vi "Timer data class VI - timer interface.vi"(8 "error in (no error)":errorcluster, 11 "Timer in":refnum<class "Timer.lvclass">) -> (0 "error out":errorcluster, 1 "counter":i8, 2 "time":string, 3 "Timer out":refnum<class "Timer.lvclass">, 5 "Milliseconds":u32)   [LabVIEW 2010, in "Timer.lvclass"]
uses:
  Timer.lvclass
  Controls/Timing Control.ctl
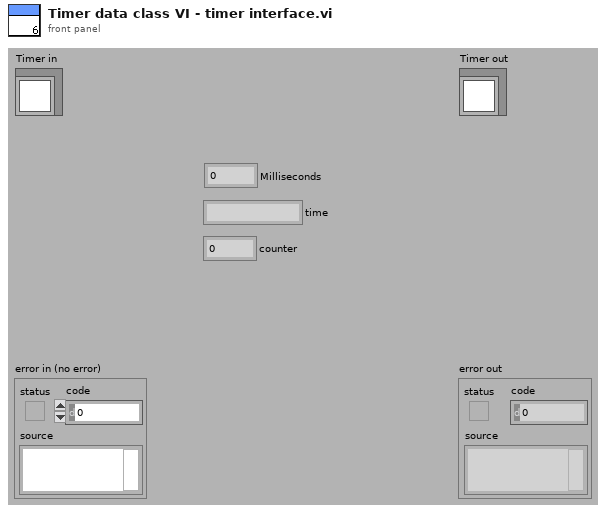
[diagram p1: front panel]
types:
  T1 = typedef "Timing Control.ctl" = enum16{"Idle", "Start", "Continue", "Reset"}
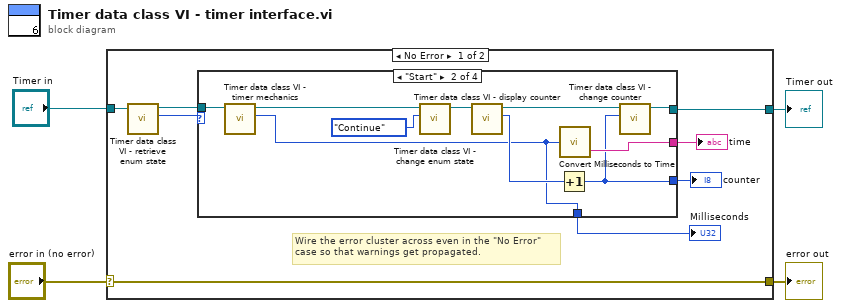
[diagram p0: block diagram]
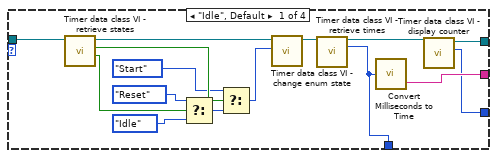
[diagram p2: hidden frame]
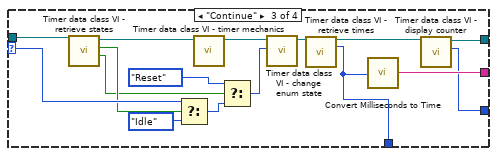
[diagram p3: hidden frame]
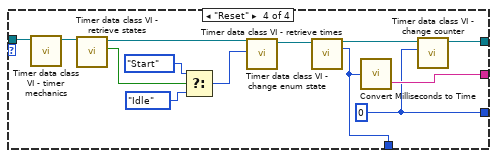
[diagram p4: hidden frame]
diagram:
  n1 = case shown="No Error" "error in (no error)" {
    selector: "error in (no error)" -> [w12 w68]
    tunnel: [w12 w68] -> w3
    tunnel: [w7 w67] -> w1
    tunnel: "Timer in" -> [w11 w67]
    frame No Error {
      # "Wire the error cluster across even in the \"No Error\"\ncase so that warnings get propagated."
      n2 = call-dynamic "Timer data class VI - retrieve enum state.vi"("Timer in"=w11) -> ("State"=w10:T1, "Timer out"=w9:refnum<class "Timer.lvclass">)  [unwired: 8 in, 1 out]
      n3 = case shown="\"Start\"" w10 {
        selector: w10 -> [_ _ w45 _]
        tunnel: w9 -> [w26 w36 w53 w66]
        tunnel: [w27 w37 w42 w60] -> w8
        tunnel: [w15 w31 w40 w56] -> w7
        tunnel: [w14 w29 w39 w55] -> w6
        tunnel: [w13 w28 w38 w54] -> w5
        frame "Idle", Default {
          n4 = call-dynamic "Timer data class VI - retrieve states.vi"("Timer in"=w26) -> ("Reset"=w21:bool, "Start/Stop"=w20:bool, "Timer out"=w25:refnum<class "Timer.lvclass">)  [unwired: 7 in, 1 out]
          n5 = Select(t=Timing_Control."Reset" ("Enum"), s=w21, f=Timing_Control."Idle" ("Enum")) -> (s? t:f=w23:T1)
          n6 = Select(t=Timing_Control."Start" ("Enum"), s=w20, f=w23) -> (s? t:f=w22:T1)
          n7 = call-dynamic "Timer data class VI - change enum state.vi"("State"=w22, "Timer in"=w25) -> ("Timer out"=w24:refnum<class "Timer.lvclass">)  [unwired: 8 in, 1 out]
          n8 = call-dynamic "Timer data class VI - retrieve times.vi"("Timer in"=w24) -> ("Timer out"=w16:refnum<class "Timer.lvclass">, "Milliseconds"=w13:u32)  [unwired: 10 in, 3 out]
          n9 = call "Convert Milliseconds to Time.vi"("milliseconds"=w13) -> ("elapsed time"=w27:string)  [unwired: 1 in]
          n10 = call "Timer data class VI - display counter.vi"("Timer in"=w16) -> ("Counter"=w14:i8, "Timer out"=w15:refnum<class "Timer.lvclass">)  [unwired: 8 in, 1 out]
        }
        frame "Start" {
          n11 = call-dynamic "Timer data class VI - timer mechanics.vi"("Timer in"=w36) -> ("elapsed time (milliseconds)"=w28:u32, "Timer out"=w35:refnum<class "Timer.lvclass">)  [unwired: 8 in, 1 out]
          n12 = call-dynamic "Timer data class VI - change enum state.vi"("State"=Timing_Control."Continue" ("Enum"), "Timer in"=w35) -> ("Timer out"=w33:refnum<class "Timer.lvclass">)  [unwired: 8 in, 1 out]
          n13 = call "Timer data class VI - display counter.vi"("Timer in"=w33) -> ("Counter"=w30:i8, "Timer out"=w32:refnum<class "Timer.lvclass">)  [unwired: 8 in, 1 out]
          n14 = Increment(x=w30) -> (x+1=w29:i8)
          n15 = call "Convert Milliseconds to Time.vi"("milliseconds"=w28) -> ("elapsed time"=w37:string)  [unwired: 1 in]
          n16 = call "Timer data class VI - change counter.vi"("Counter"=w29, "Timer in"=w32) -> ("Timer out"=w31:refnum<class "Timer.lvclass">)  [unwired: 8 in, 1 out]
        }
        frame "Continue" {
          n17 = call-dynamic "Timer data class VI - retrieve states.vi"("Timer in"=w53) -> ("Reset"=w43:bool, "Start/Stop"=w44:bool, "Timer out"=w46:refnum<class "Timer.lvclass">)  [unwired: 7 in, 1 out]
          n18 = Select(t=w45, s=w44, f=enum16{"Idle", "Start", "Continue", "Reset"}."Idle" ("Enum")) -> (s? t:f=w51:T1)
          n19 = call-dynamic "Timer data class VI - timer mechanics.vi"("Timer in"=w46) -> ("Timer out"=w48:refnum<class "Timer.lvclass">)  [unwired: 8 in, 2 out]
          n20 = Select(t=enum16{"Idle", "Start", "Continue", "Reset"}."Reset" ("Enum"), s=w43, f=w51) -> (s? t:f=w49:T1)
          n21 = call-dynamic "Timer data class VI - change enum state.vi"("State"=w49, "Timer in"=w48) -> ("Timer out"=w47:refnum<class "Timer.lvclass">)  [unwired: 8 in, 1 out]
          n22 = call-dynamic "Timer data class VI - retrieve times.vi"("Timer in"=w47) -> ("Timer out"=w41:refnum<class "Timer.lvclass">, "Milliseconds"=w38:u32)  [unwired: 10 in, 3 out]
          n23 = call "Convert Milliseconds to Time.vi"("milliseconds"=w38) -> ("elapsed time"=w42:string)  [unwired: 1 in]
          n24 = call "Timer data class VI - display counter.vi"("Timer in"=w41) -> ("Counter"=w39:i8, "Timer out"=w40:refnum<class "Timer.lvclass">)  [unwired: 8 in, 1 out]
        }
        frame "Reset" {
          w55 = i8 0 ("Counter")
          n25 = call-dynamic "Timer data class VI - timer mechanics.vi"("Timer in"=w66) -> ("Timer out"=w64:refnum<class "Timer.lvclass">)  [unwired: 8 in, 2 out]
          n26 = call-dynamic "Timer data class VI - retrieve states.vi"("Timer in"=w64) -> ("Start/Stop"=w63:bool, "Timer out"=w61:refnum<class "Timer.lvclass">)  [unwired: 7 in, 2 out]
          n27 = Select(t=Timing_Control."Start" ("Enum"), s=w63, f=Timing_Control."Idle" ("Enum")) -> (s? t:f=w62:T1)
          n28 = call-dynamic "Timer data class VI - change enum state.vi"("State"=w62, "Timer in"=w61) -> ("Timer out"=w65:refnum<class "Timer.lvclass">)  [unwired: 8 in, 1 out]
          n29 = call-dynamic "Timer data class VI - retrieve times.vi"("Timer in"=w65) -> ("Timer out"=w57:refnum<class "Timer.lvclass">, "Milliseconds"=w54:u32)  [unwired: 10 in, 3 out]
          n30 = call "Convert Milliseconds to Time.vi"("milliseconds"=w54) -> ("elapsed time"=w60:string)  [unwired: 1 in]
          n31 = call "Timer data class VI - change counter.vi"("Counter"=w55, "Timer in"=w57) -> ("Timer out"=w56:refnum<class "Timer.lvclass">)  [unwired: 8 in, 1 out]
        }
      }
      "time" <- w8
      "counter" <- w6
      "Milliseconds" <- w5
    }
    frame Error {
    }
  }
  "error out" <- w3
  "Timer out" <- w1
